vi "CAN Konfig.vi"() -> ()   [LabVIEW 2020]
uses:
  195161_2023-03-15/Allgemein/allgemeine Sub-VIs.lvlib
  195161_2023-03-15/cRIO/CAN Interface/CAN Interface.lvlib
  FGV CAN Daten Aktionen.ctl
  Baude Rate.ctl
  <vilib>/xnet/xnet.llb/XNET Frame Type CAN.ctl
  <vilib>/xnet/xnet.llb/XNET Frame CAN.ctl
  Visualisierungs Elemente/Button.ctl
panel:
  in  "Zahlen Anzeige:":enum16{"dezimal", "hexadezimal"}(ring)
  in  "Frame-ID GPS:":u32=512
  in  "Frame-ID Semtech:":u32=890
  in  "Frame-ID Pegasor 3:":u32=980
  in  "Frame-ID Pegasor 2:":u32=970
  in  "Frame-ID Pegasor 1:":u32=960
  in  "Frame-ID Statuswerte:":u32=990
  in  "Frame-ID MS 3:":u32=950
  in  "Frame-ID MS 2:":u32=940
  in  "Frame-ID MS 1:":u32=930
  in  "Frame-ID FT-IR 3:":u32=920
  in  "Frame-ID FT-IR 2:":u32=910
  in  "Frame-ID FT-IR 1:":u32=900 format="%.0x"
  in  "Baude Rate:":T1=250000 items=["40 kBaud"=40000, "50 kBaud"=50000, "62,5 kBaud"=62500, "80 kBaud"=80000, "83,3 kBaud"=83300, "100 kBaud"=100000, "125 kBaud"=125000, "160 kBaud"=160000, "200 kBaud"=200000, "250 kBaud"=250000, "400 kBaud"=400000, "500 kBaud"=500000, "800 kBaud"=800000, "1 MBaud"=1000000]
  in  "CAN Cluster:":refnum<k21>="06X-52T2_171214"
  in  "Select Interface:":refnum<k21>="CAN1"
  in  "Speichern":T2
  out "data":T3[](array[typedef])=[{"timestamp"=timestamp(0 s since 1904-01-01), "payload"=[0, 2, 3, 4, 5, 6, 7, 8], "identifier"=2, "type"=0, "extended?"=FALSE, "echo?"=FALSE}, {"timestamp"=timestamp(0 s since 1904-01-01), "payload"=[0, 1, 2, 3, 4, 5, 6, 7], "identifier"=3, "type"=0, "extended?"=FALSE, "echo?"=FALSE}] {"payload" format="%x"; "timestamp" format="%<%.7X\n%x>T"; "type" items=["CAN Data"=0, "CAN Remote"=1, "CAN Bus Error"=2, "CAN 2.0 Data"=8, "CAN FD Data"=16, "CAN FD+BRS Data"=24, "J1939 Data"=192, "Delay"=224, "Log Trigger"=225, "Start Trigger"=226]; "identifier" format="%x"}
  # "CAN Konfig"
  # "CAN Status (Daten)"
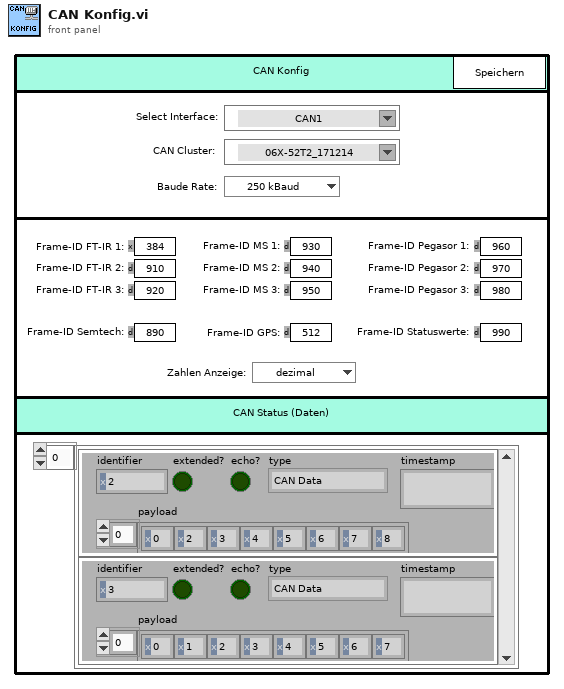
[diagram p1: front panel]
types:
  T1 = typedef "CAN Interface.lvlib/Baude Rate.ctl" = u32
  T2 = typedef "Button.ctl" = bool
  T3 = typedef "XNET Frame CAN.ctl" = cluster{"timestamp":timestamp, "payload":u8[], "identifier":u32, "type":T4, "extended?":bool, "echo?":bool}
  T4 = typedef "XNET Frame Type CAN.ctl" = u8
  T5 = typedef "CAN Interface.lvlib/FGV CAN Daten Aktionen.ctl" = enum16{"lesen", "Daten", "Konfig", "laden", "speichern", "Status"}
  T6 = typedef "CAN Konfig.lvlib/Konfig Daten PC.ctl" = cluster{"Baude Rate":T1, "COM state":u8, "Frame-ID FTIR Start":u32, "Frame-ID FTIR End":u32, "Frame-ID Status Start":u32, "Frame-ID Status End":u32, "Zustand Information":u32, "Aktion":u32, "Frame-ID FTIR Arry":u32[], "Frame-ID Status Arry":u32[], "GPS Start":u32, "Interface":refnum<k21>}
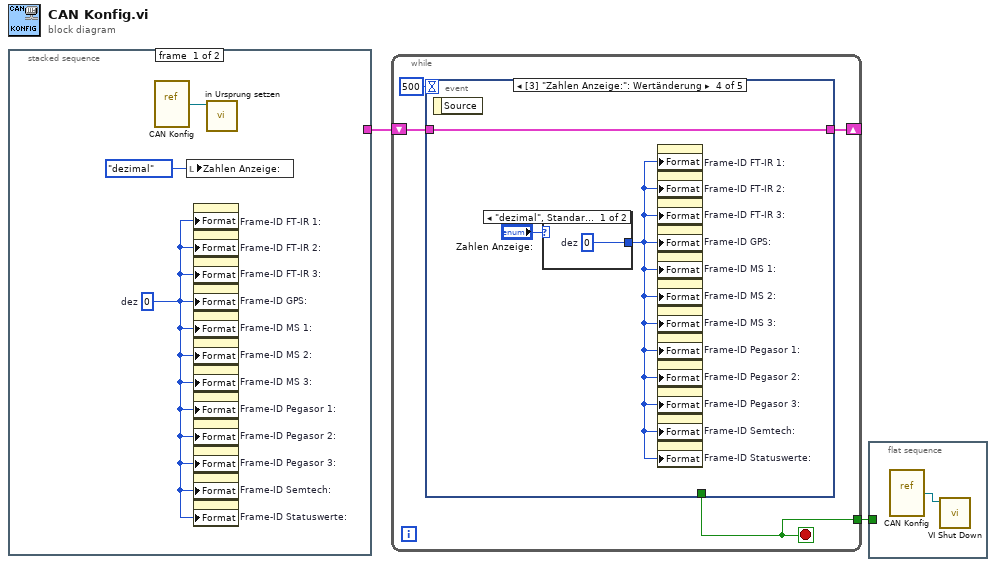
[diagram p0: block diagram]
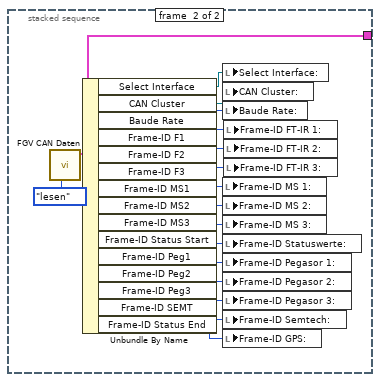
[diagram p2: hidden frame]
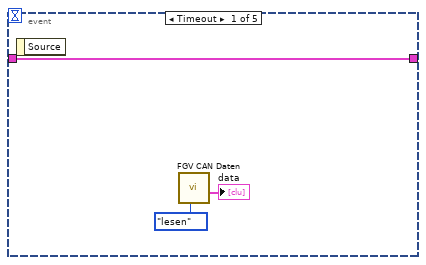
[diagram p3: hidden frame]
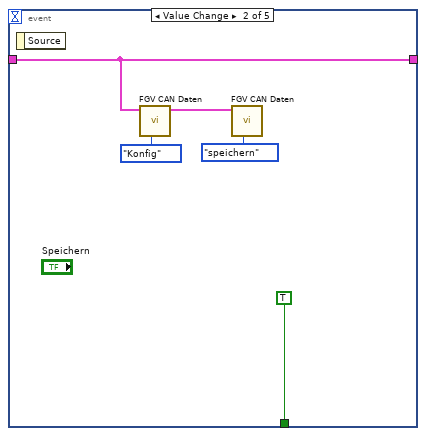
[diagram p4: hidden frame]
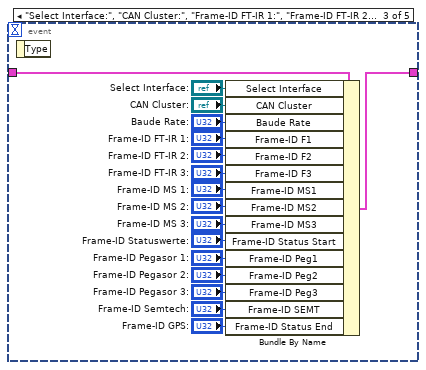
[diagram p5: hidden frame]
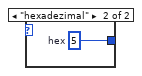
[diagram p6: hidden frame]
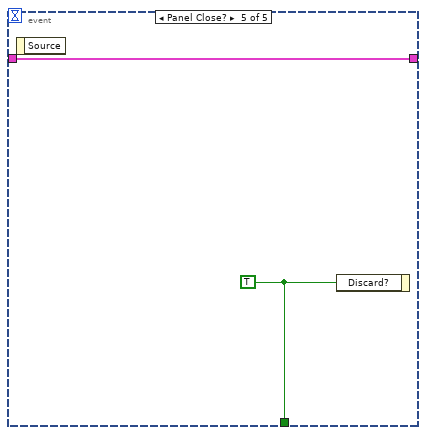
[diagram p7: hidden frame]
diagram:
  n1 = stacked-sequence {
    tunnel: [_ w11] -> w1
    frame #0 {
      w4 = u8 0  # dez
      n2 = vi-ref "CAN Konfig.vi"() -> (w5:refnum<vi>)
      n3 = local write "Zahlen Anzeige:"(enum16{"dezimal", "hexadezimal"}."dezimal" ("Zahlen Anzeige:")) -> ()
      n4 = property on="Frame-ID FT-IR 1:" class="DigWert (strikt)"("Format"=w4) -> ()  [unwired: 2 in, 2 out]
      n5 = property on="Frame-ID FT-IR 2:" class="DigWert (strikt)"("Format"=w4) -> ()  [unwired: 2 in, 2 out]
      n6 = property on="Frame-ID FT-IR 3:" class="DigWert (strikt)"("Format"=w4) -> ()  [unwired: 2 in, 2 out]
      n7 = property on="Frame-ID GPS:" class="DigWert (strikt)"("Format"=w4) -> ()  [unwired: 2 in, 2 out]
      n8 = property on="Frame-ID MS 1:" class="DigWert (strikt)"("Format"=w4) -> ()  [unwired: 2 in, 2 out]
      n9 = property on="Frame-ID MS 2:" class="DigWert (strikt)"("Format"=w4) -> ()  [unwired: 2 in, 2 out]
      n10 = property on="Frame-ID MS 3:" class="DigWert (strikt)"("Format"=w4) -> ()  [unwired: 2 in, 2 out]
      n11 = property on="Frame-ID Pegasor 1:" class="DigWert (strikt)"("Format"=w4) -> ()  [unwired: 2 in, 2 out]
      n12 = property on="Frame-ID Pegasor 2:" class="DigWert (strikt)"("Format"=w4) -> ()  [unwired: 2 in, 2 out]
      n13 = property on="Frame-ID Pegasor 3:" class="DigWert (strikt)"("Format"=w4) -> ()  [unwired: 2 in, 2 out]
      n14 = property on="Frame-ID Semtech:" class="DigWert (strikt)"("Format"=w4) -> ()  [unwired: 2 in, 2 out]
      n15 = property on="Frame-ID Statuswerte:" class="DigWert (strikt)"("Format"=w4) -> ()  [unwired: 2 in, 2 out]
      n16 = call "in Ursprung setzen.vi"("VI Referenz"=w5) -> ()  [unwired: 11 in]
    }
    frame #1 {
      n17 = call "FGV CAN Daten.vi"("Aktionen"=FGV_CAN_Daten_Aktionen."lesen") -> ("Konfig Daten"=w11:T6)  [unwired: 8 in, 2 out]
      n18 = Unbundle By Name(w11) -> ("Select Interface"=w21:refnum<k21>, "CAN Cluster"=w20:refnum<k21>, "Baude Rate"=w19:T1, "Frame-ID F1"=w18:u32, "Frame-ID F2"=w17:u32, "Frame-ID F3"=w16:u32, "Frame-ID MS1"=w15:u32, "Frame-ID MS2"=w14:u32, "Frame-ID MS3"=w13:u32, "Frame-ID Status Start"=w12:u32, "Frame-ID Peg1"=w10:u32, "Frame-ID Peg2"=w9:u32, "Frame-ID Peg3"=w8:u32, "Frame-ID SEMT"=w7:u32, "Frame-ID Status End"=w6:u32)
      n19 = local write "Select Interface:"(w21) -> ()
      n20 = local write "CAN Cluster:"(w20) -> ()
      n21 = local write "Baude Rate:"(w19) -> ()
      n22 = local write "Frame-ID MS 1:"(w15) -> ()
      n23 = local write "Frame-ID MS 2:"(w14) -> ()
      n24 = local write "Frame-ID MS 3:"(w13) -> ()
      n25 = local write "Frame-ID Statuswerte:"(w12) -> ()
      n26 = local write "Frame-ID Pegasor 1:"(w10) -> ()
      n27 = local write "Frame-ID Pegasor 2:"(w9) -> ()
      n28 = local write "Frame-ID Pegasor 3:"(w8) -> ()
      n29 = local write "Frame-ID Semtech:"(w7) -> ()
      n30 = local write "Frame-ID GPS:"(w6) -> ()
      n31 = local write "Frame-ID FT-IR 1:"(w18) -> ()
      n32 = local write "Frame-ID FT-IR 2:"(w17) -> ()
      n33 = local write "Frame-ID FT-IR 3:"(w16) -> ()
    }
  }
  n34 = while {
    tunnel: [w25] -> w2
    shift-right: [w23] -> _
    shift-left: w1 -> [w24]
    stop <- w25 stop-if-true
    n35 = event shown="[3] \"Zahlen Anzeige:\": Wertänderung" {
      selector: _ -> [_ _ _ _ _]
      dyn-events: _ -> [_ _ _ _ _]
      timeout: 500 -> [_ _ _ _ _]
      tunnel: [_ TRUE ("Verwerfen?") _ _ w58] -> w25
      tunnel: w24 -> [w27 w30 w40 w54 w57]
      tunnel: [w27 w30 w41 w54 w57] -> w23
      event Timeout {
        n36 = event-data() -> ()  [unwired: 1 in, 1 out]
        n37 = call "FGV CAN Daten.vi"("Aktionen"=FGV_CAN_Daten_Aktionen."lesen") -> ("data"=→"data":T3[])  [unwired: 8 in, 2 out]
      }
      event Value Change {
        n38 = event-data() -> ()  [unwired: 1 in, 1 out]
        n39 = call "FGV CAN Daten.vi"("Aktionen"=FGV_CAN_Daten_Aktionen."Konfig", "Konfig Daten 2"=w30) -> ("Konfig Daten"=w31:T6)  [unwired: 7 in, 2 out]
        n40 = call "FGV CAN Daten.vi"("Aktionen"=FGV_CAN_Daten_Aktionen."speichern", "Konfig Daten 2"=w31) -> ()  [unwired: 7 in, 3 out]
      }
      event "Select Interface:", "CAN Cluster:", "Frame-ID FT-IR 1:", "Frame-ID FT-IR 2:", "Frame-ID FT-IR 3:", "Frame-ID MS 1:", "Frame-ID MS 2:", "Frame-ID MS 3:", "Frame-ID Statuswerte:", "Frame-ID Pegasor 1:", "Frame-ID Pegasor 2:", "Frame-ID Pegasor 3:", "Frame-ID Semtech:", "Frame-ID GPS:": Value Change {
        n41 = event-data() -> ()  [unwired: 1 in, 1 out]
        n42 = Bundle By Name(cluster=w40, "Select Interface"="Select Interface:", "CAN Cluster"="CAN Cluster:", "Baude Rate"="Baude Rate:", "Frame-ID F1"="Frame-ID FT-IR 1:", "Frame-ID F2"="Frame-ID FT-IR 2:", "Frame-ID F3"="Frame-ID FT-IR 3:", "Frame-ID MS1"="Frame-ID MS 1:", "Frame-ID MS2"="Frame-ID MS 2:", "Frame-ID MS3"="Frame-ID MS 3:", "Frame-ID Status Start"="Frame-ID Statuswerte:", "Frame-ID Peg1"="Frame-ID Pegasor 1:", "Frame-ID Peg2"="Frame-ID Pegasor 2:", "Frame-ID Peg3"="Frame-ID Pegasor 3:", "Frame-ID SEMT"="Frame-ID Semtech:", "Frame-ID Status End"="Frame-ID GPS:") -> (w41:T6)
      }
      event "Zahlen Anzeige:": Value Change {
        n43 = event-data() -> ()  [unwired: 1 in, 1 out]
        n44 = case shown="\"dezimal\", Standard" "Zahlen Anzeige:" {
          tunnel: [w55 w56] -> w53
          frame "dezimal", Default {
            w55 = u8 0  # dez
          }
          frame "hexadezimal" {
            w56 = u8 5  # hex
          }
        }
        n45 = property on="Frame-ID FT-IR 1:" class="DigWert (strikt)"("Format"=w53) -> ()  [unwired: 2 in, 2 out]
        n46 = property on="Frame-ID FT-IR 2:" class="DigWert (strikt)"("Format"=w53) -> ()  [unwired: 2 in, 2 out]
        n47 = property on="Frame-ID FT-IR 3:" class="DigWert (strikt)"("Format"=w53) -> ()  [unwired: 2 in, 2 out]
        n48 = property on="Frame-ID GPS:" class="DigWert (strikt)"("Format"=w53) -> ()  [unwired: 2 in, 2 out]
        n49 = property on="Frame-ID MS 1:" class="DigWert (strikt)"("Format"=w53) -> ()  [unwired: 2 in, 2 out]
        n50 = property on="Frame-ID MS 2:" class="DigWert (strikt)"("Format"=w53) -> ()  [unwired: 2 in, 2 out]
        n51 = property on="Frame-ID MS 3:" class="DigWert (strikt)"("Format"=w53) -> ()  [unwired: 2 in, 2 out]
        n52 = property on="Frame-ID Pegasor 1:" class="DigWert (strikt)"("Format"=w53) -> ()  [unwired: 2 in, 2 out]
        n53 = property on="Frame-ID Pegasor 2:" class="DigWert (strikt)"("Format"=w53) -> ()  [unwired: 2 in, 2 out]
        n54 = property on="Frame-ID Pegasor 3:" class="DigWert (strikt)"("Format"=w53) -> ()  [unwired: 2 in, 2 out]
        n55 = property on="Frame-ID Semtech:" class="DigWert (strikt)"("Format"=w53) -> ()  [unwired: 2 in, 2 out]
        n56 = property on="Frame-ID Statuswerte:" class="DigWert (strikt)"("Format"=w53) -> ()  [unwired: 2 in, 2 out]
      }
      event Panel Close? {
        w58 = TRUE ("Verwerfen?")
        n57 = event-data() -> ()  [unwired: 1 in, 1 out]
        n58 = event-data("Discard?"=w58) -> ()  [unwired: 1 in, 1 out]
      }
    }
  }
  n59 = flat-sequence {
    tunnel: w2 -> [_]
    frame #0 {
      n60 = vi-ref "CAN Konfig.vi"() -> (w59:refnum<vi>)
      n61 = call "VI Shut Down.vi"("VI Referenz"=w59) -> ()  [unwired: 11 in]
    }
  }
